vi "Vending Timer.vi"(5 "Set/Get":enum16{"Get Timer", "Set Timer"}(ring), 6 "Error In":errorcluster, 9 "Target Time":dbl) -> (0 "Error Out":errorcluster, 2 "Elapsed Time":dbl, 3 "Elapsed?":bool)   [LabVIEW 2019]
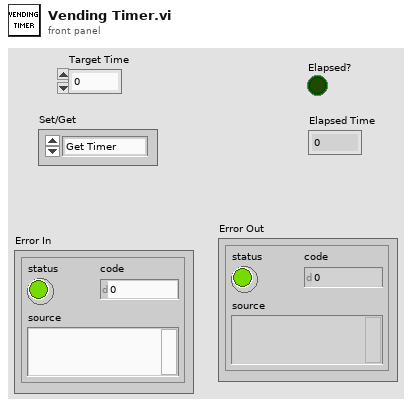
[diagram p1: front panel]
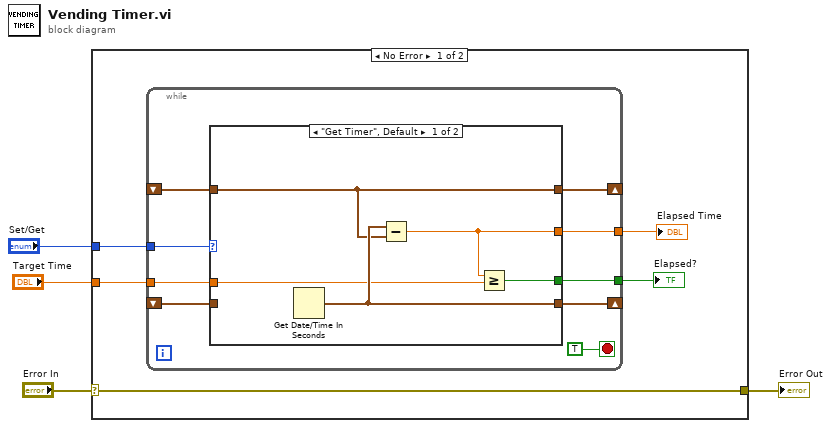
[diagram p0: block diagram]
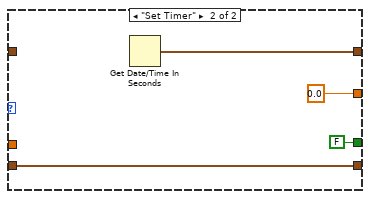
[diagram p2: hidden frame]
diagram:
  n1 = case shown="No Error" "Error In" {
    selector: "Error In" -> [w5 w28]
    tunnel: [w5 w28] -> w3
    tunnel: "Set/Get" -> [w9 _]
    tunnel: "Target Time" -> [w7 _]
    frame No Error {
      n2 = while {
        shift-right: [w18] -> _
        shift-left: _ -> [w16]
        tunnel: w9 -> [w17]
        shift-right: [w15] -> _
        shift-left: _ -> [w14]
        tunnel: [w13] -> w8
        tunnel: w7 -> [w11]
        tunnel: [w10] -> w6
        stop <- TRUE stop-if-true
        n3 = case shown="\"Get Timer\", Default" w17 {
          tunnel: [w22 w27] -> w18
          tunnel: w16 -> [w22 _]
          tunnel: [w23 w26] -> w15
          tunnel: w14 -> [_ w26]
          tunnel: [w19 0.0] -> w13
          tunnel: w11 -> [w21 _]
          tunnel: [w20 FALSE] -> w10
          frame "Get Timer", Default {
            n4 = Get Date/Time In Seconds() -> (seconds since 1Jan1904=w23:timestamp)
            n5 = Subtract(x=w23, y=w22) -> (x-y=w19:dbl)
            n6 = Greater Or Equal?(x=w19, y=w21) -> (x >= y?=w20:bool)
          }
          frame "Set Timer" {
            n7 = Get Date/Time In Seconds() -> (seconds since 1Jan1904=w27:timestamp)
          }
        }
      }
      "Elapsed Time" <- w8
      "Elapsed?" <- w6
    }
    frame Error {
    }
  }
  "Error Out" <- w3
